vi "解析交互信息.vi"(2 "交互信息":string) -> (5 "提示":string[](array[string]), 6 "备选信息":string[][](array[string]), 7 "补充信息":string[](array[string]))   [LabVIEW 2018]
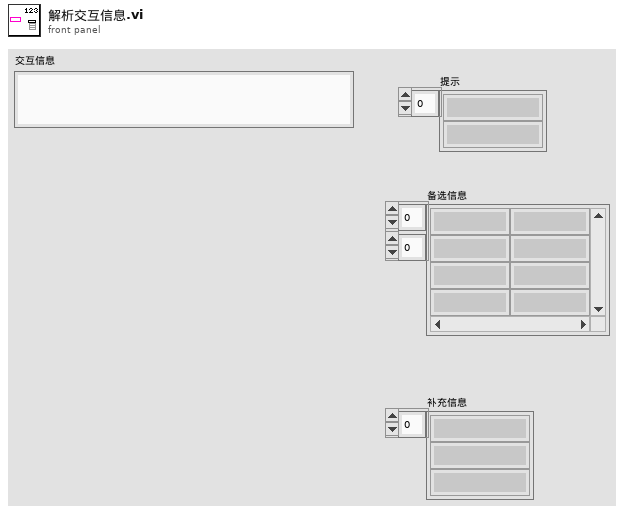
[diagram p1: front panel]
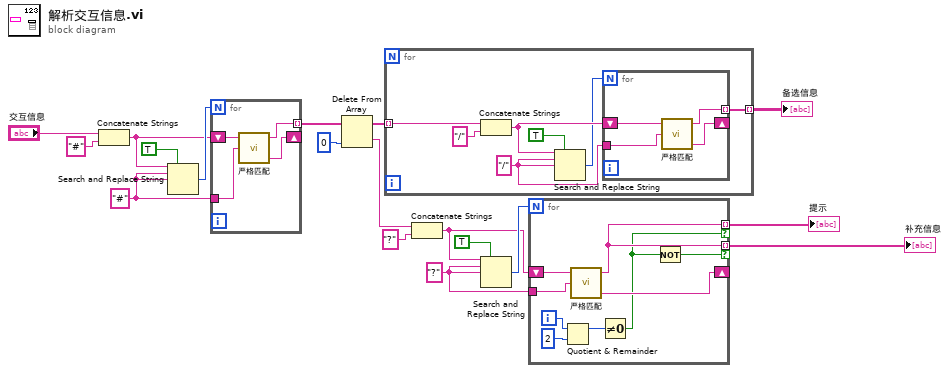
[diagram p0: block diagram]
diagram:
  w11 = "?" ("搜索字符串")
  w17 = "#" ("搜索字符串")
  n1 = Concatenate Strings("交互信息", "#" ("字符串")) -> (w13:string)
  n2 = Search and Replace String(replace all?=TRUE ("忽略大小写？(F)"), input string=w13, search string=w17, replace string=w17) -> (number of replacements=w18:i32)  [unwired: 4 in, 3 out]
  n3 = for {
    N: w18 -> [_]
    shift-right: [w21] -> _
    shift-left: w13 -> [w22]
    tunnel: [w20] -> w5 mode=indexing
    tunnel: w17 -> [w19]
    n4 = call "严格匹配.vi"("搜索字符串"=w19, "输入字符串"=w22) -> ("之后"=w21:string, "之前"=w20:string)  [unwired: 1 in, 1 out]
  }
  n5 = Delete From Array(array=w5, index=0 ("索引")) -> (deleted portion=w9:string, array with subset deleted=w4:string[])  [unwired: 1 in]
  n6 = for {
    tunnel: w4 -> [w24] mode=indexing
    tunnel: [w23] -> w2 mode=indexing
    w26 = "/" ("搜索字符串")
    n7 = Concatenate Strings(w24, "/" ("字符串")) -> (w28:string)
    n8 = Search and Replace String(replace all?=TRUE ("忽略大小写？(F)"), input string=w28, search string=w26, replace string=w26) -> (number of replacements=w27:i32)  [unwired: 4 in, 3 out]
    n9 = for {
      N: w27 -> [_]
      shift-right: [w32] -> _
      shift-left: w28 -> [w33]
      tunnel: [w31] -> w23 mode=indexing
      tunnel: w26 -> [w30]
      n10 = call "严格匹配.vi"("搜索字符串"=w30, "输入字符串"=w33) -> ("之后"=w32:string, "之前"=w31:string)  [unwired: 1 in, 1 out]
    }
  }
  "备选信息" <- w2
  n11 = Concatenate Strings(w9, "?" ("字符串")) -> (w8:string)
  n12 = Search and Replace String(replace all?=TRUE ("忽略大小写？(F)"), input string=w8, search string=w11, replace string=w11) -> (number of replacements=w10:i32)  [unwired: 4 in, 3 out]
  n13 = for {
    N: w10 -> [_]
    shift-right: [w41] -> _
    shift-left: w8 -> [w42]
    tunnel: [w36] -> w3 mode=indexing if=w35
    tunnel: w11 -> [w40]
    tunnel: [w36] -> w1 mode=indexing if=w34
    i -> [w39]
    n14 = Quotient & Remainder(x=w39, y=2) -> (x-y*floor(x/y)=w37:i32)  [unwired: 1 out]
    n15 = call "严格匹配.vi"("搜索字符串"=w40, "输入字符串"=w42) -> ("之后"=w41:string, "之前"=w36:string)  [unwired: 1 in, 1 out]
    n16 = Not Equal To 0?(x=w37) -> (x != 0?=w35:bool)
    n17 = Not(x=w35) -> (.not. x?=w34:bool)
  }
  "提示" <- w3
  "补充信息" <- w1
